vi "Read_Characters_From_File.ph.vi"(0 "file path (dialog if empty)":path, 2 "number of characters (all:-1)":i32=-1, 3 "start of read offset (chars.: 0)":i32, 5 "convert eol? (no:F)":bool) -> (6 "new file path (NotAPath if cancelled)":path, 7 "character string":string, 8 "EOF?":bool, 9 "mark after read (chars.)":i32)   [LabVIEW 2010]
doc: "Reads a specified number of characters from a byte stream file beginning at a specified character offset. The VI opens the file beforehand and closes it afterwards.\n\nfile path is the path name of the file. If file path is empty (default value) or is Not A Path, the VI displays a File dialog box from which you can select a file. Error 43 occurs if the user cancels the dialog. \n\nnumber of character is the maximum number of characters the VI reads. The VI reads fewer characters if it reaches the EOF first. The default value is -1 characters, which means to read the entire file.\n\nstart of read offset is the position in the file, measured in characters (or bytes), at which the VI begins reading.\n\nnew file path is the path of the file from which the VI read data. You can use this output to determine the path of a file that you open using dialog. new file path returns Not A Path if the user selects Cancel from the dialog box.\n\ncharacters string is the data read from the file\n\nmark after read is the location of the file mark after the read; it points to the character in the file following the last character read.\n\nEOF? is TRUE if you attempt to read past the end of file."
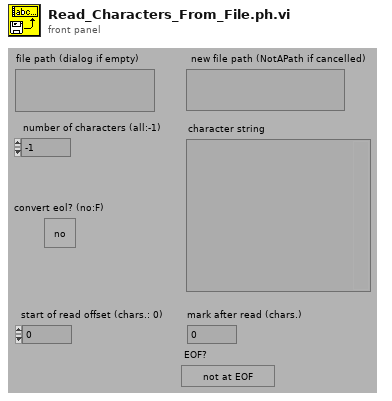
[diagram p1: front panel]
types:
  T1 = typedef "File_Status.ctl" = enum16{"Invalid Path", "This is a folder pathname", "Generic File Error", "Directory structure cannot be created", "File cannot be created", "File can be created", "File exist but read only", "File exist but no access", "File exist with read and write access"}
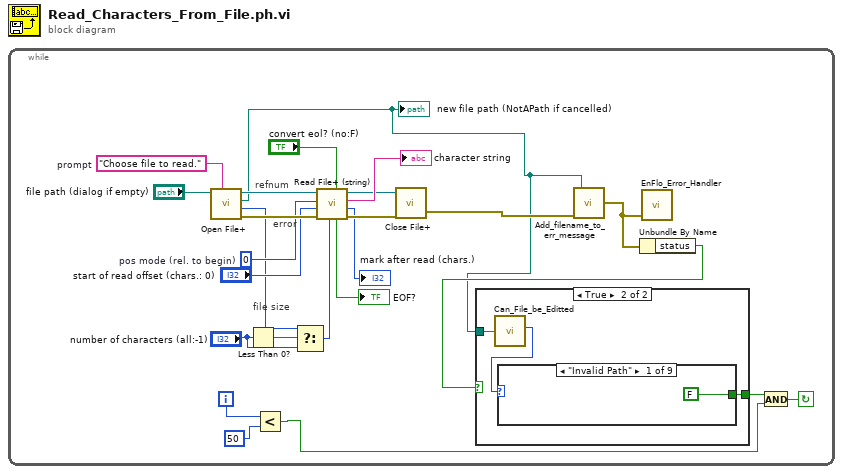
[diagram p0: block diagram]
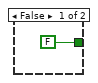
[diagram p2: hidden frame]
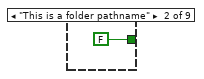
[diagram p3: hidden frame]
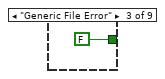
[diagram p4: hidden frame]
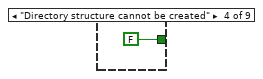
[diagram p5: hidden frame]
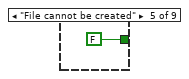
[diagram p6: hidden frame]
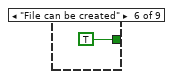
[diagram p7: hidden frame]
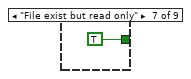
[diagram p8: hidden frame]
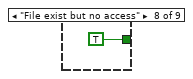
[diagram p9: hidden frame]
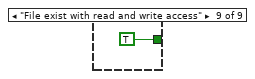
[diagram p10: hidden frame]
diagram:
  n1 = while {
    i -> [w5]
    stop <- w1 continue-if-true
    w23 = i16 0  # pos mode (rel. to begin)
    w18 = "Choose file to read."  # prompt
    # "file size"
    # "error"
    # "refnum"
    n2 = call <vilib>:"Open File+.vi"("prompt"=w18, "file path (\" \")"="file path (dialog if empty)") -> ("error out"=w25:errorcluster, "file size (bytes)"=w14:i32, "file path"=w6:path, "refnum"=w16:refnum<file>)  [unwired: 4 in, 2 out]
    "new file path (NotAPath if cancelled)" <- w6
    n3 = Less Than 0?(x="number of characters (all:-1)") -> (x < 0?=w15:bool)
    n4 = Less?(x=w5, y=50) -> (x < y?=w2:bool)
    n5 = Select(t=w14, s=w15, f="number of characters (all:-1)") -> (s? t:f=w12:i32)
    n6 = call <vilib>:"Read File+ (string).vi"("convert eol? (no:F)"="convert eol? (no:F)", "count"=w12, "error in (no error)"=w25, "pos offset (bytes:0)"="start of read offset (chars.: 0)", "pos mode (rel. to current:2)"=w23, "refnum"=w16) -> ("error out"=w21:errorcluster, "mark after read (bytes)"=→"mark after read (chars.)":i32, "string"=→"character string":string, "dup refnum"=w20:refnum<file>, "EOF?"=→"EOF?":bool)  [unwired: 1 out]
    n7 = call <vilib>:"Close File+.vi"("error in (no error)"=w21, "refnum"=w20) -> ("error out"=w10:errorcluster)  [unwired: 5 out]
    n8 = call "Add_filename_to_err_message.vi"("error in (no error)"=w10, "Path"=w6) -> ("error out"=w8:errorcluster)
    n9 = Unbundle By Name(w8) -> ("status"=w7:bool)
    n10 = case shown="True" w7 {
      tunnel: w6 -> [_ w29]
      tunnel: [FALSE w27] -> w3
      frame False {
      }
      frame True {
        n11 = call "Can_File_be_Editted.vi"("Filename"=w29) -> ("File Status"=w28:T1)  [unwired: 3 out]
        n12 = case shown="\"Invalid Path\"" w28 {
          tunnel: [FALSE FALSE FALSE FALSE FALSE TRUE TRUE TRUE TRUE] -> w27
          frame "Invalid Path" {
          }
          frame "This is a folder pathname" {
          }
          frame "Generic File Error" {
          }
          frame "Directory structure cannot be created" {
          }
          frame "File cannot be created" {
          }
          frame "File can be created" {
          }
          frame "File exist but read only" {
          }
          frame "File exist but no access" {
          }
          frame "File exist with read and write access" {
          }
        }
      }
    }
    n13 = call "EnFlo_Error_Handler.vi"("error in (no error)"=w8) -> ()  [unwired: 2 in, 3 out]
    n14 = And(x=w3, y=w2) -> (x .and. y?=w1:bool)
  }
